vi "1.- FGV Serial.vi"(7 "VISA resource name":refnum<visa-resource-name>="COM3", 8 "error in (no error)":errorcluster, 10 "Command":string="H", 11 "Task":T1) -> (0 "error out":errorcluster, 2 "Receive buffer":string, 3 "return count":u32)   [LabVIEW 2014]
uses:
  control/FGV Serial Tasks.ctl
  <vilib>/Instr/_visa.llb/VISA Flush IO Buffer Mask.ctl
  <vilib>/Instr/_visa.llb/VISA Configure Serial Port (Instr).vi
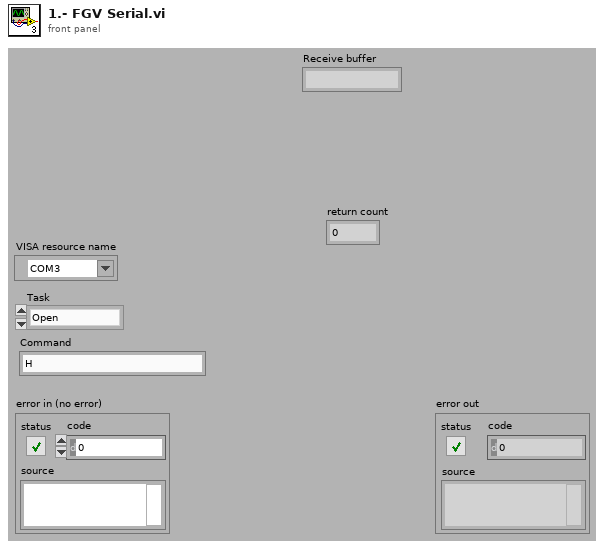
[diagram p1: front panel]
types:
  T1 = typedef "FGV Serial Tasks.ctl" = enum16{"Open", "Read", "Write", "Close", "Flush"}
  T2 = typedef "VISA Flush IO Buffer Mask.ctl" = u16
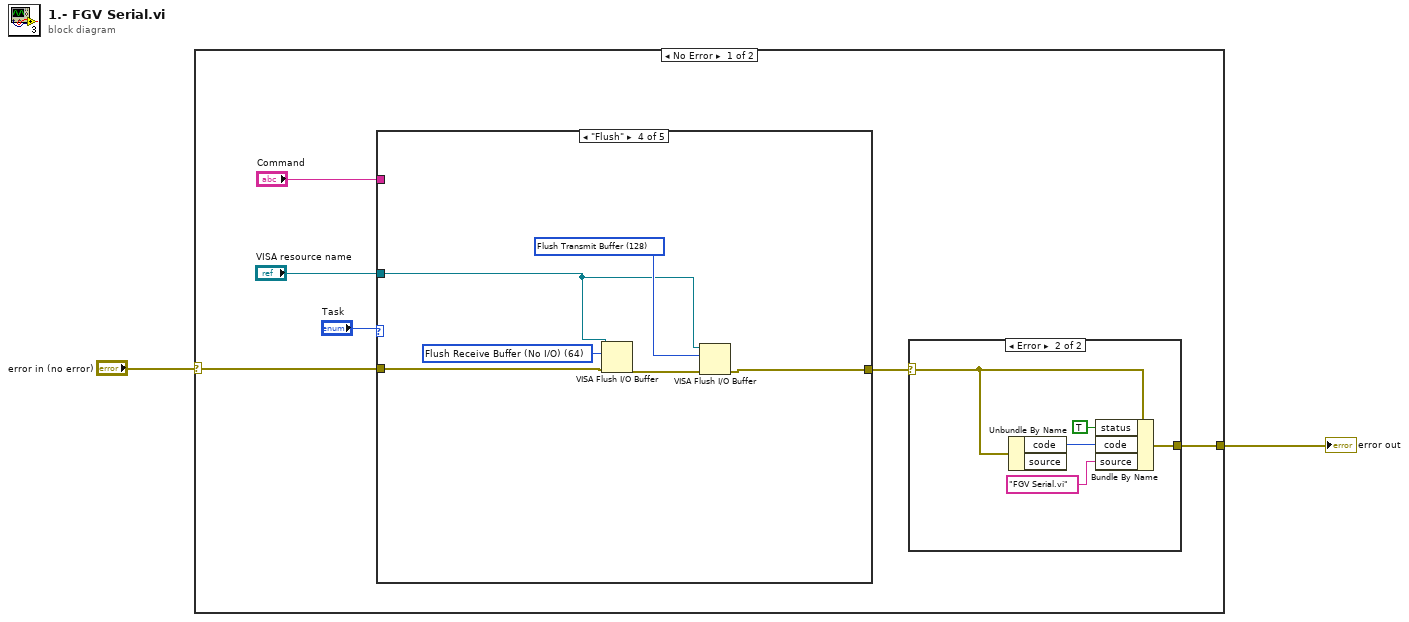
[diagram p0: block diagram]
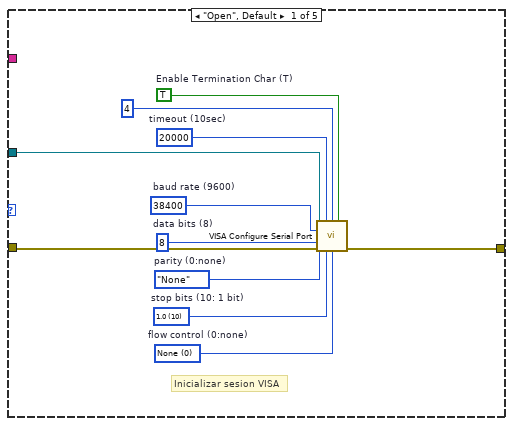
[diagram p3: hidden frame]
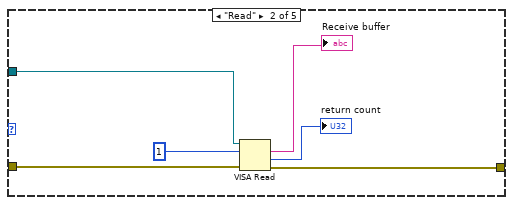
[diagram p4: hidden frame]
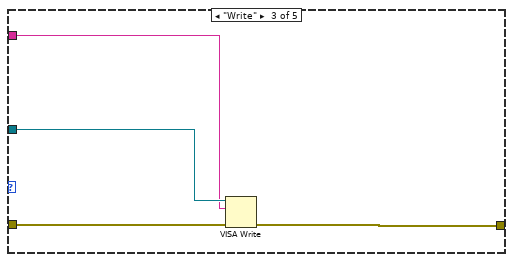
[diagram p5: hidden frame]
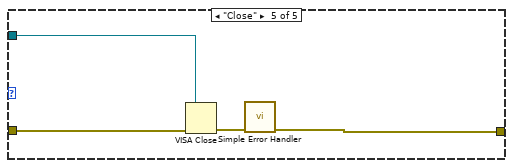
[diagram p6: hidden frame]
diagram:
  n1 = case shown="No Error" "error in (no error)" {
    selector: "error in (no error)" -> [w7 w46]
    tunnel: [w3 w46] -> w1
    frame No Error {
      n2 = case shown="\"Flush\"" "Task" {
        tunnel: "VISA resource name" -> [w18 w28 w33 w38 w42]
        tunnel: [w17 w31 w34 w36 w43] -> w4
        tunnel: w7 -> [w16 w27 w35 w41 w44]
        tunnel: "Command" -> [_ _ w32 _ _]
        frame "Open", Default {
          w23 = u16 0 items=["None", "XON/XOFF", "RTS/CTS", "XON/XOFF & RTS/CTS", "DTR/DSR", "XON/XOFF & DTR/DSR"]  # flow control (0:none)
          w22 = u16 10 items=["1.0"=10, "1.5"=15, "2.0"=20]  # stop bits (10: 1 bit)
          w21 = enum16{"None", "Odd", "Even", "Mark", "Space"}."None"  # parity (0:none)
          w20 = u16 8  # data bits (8)
          w19 = u32 38400  # baud rate (9600)
          w24 = u32 20000  # timeout (10sec)
          w25 = TRUE  # Enable Termination Char (T)
          # "Inicializar sesion VISA"
          n3 = call-poly "VISA Configure Serial Port"("VISA resource name"=w18, "timeout (10sec)"=w24, "termination char\n(0xA = '\\n' = LF)"=u8 4 ("termination char\n(0xA = '\\n' = LF)"), "Enable Termination\nChar (T)"=w25, "baud rate (9600)"=w19, "data bits (8)"=w20, "parity (0:none)"=w21, "error in (no error)"=w16, "stop bits (10: 1 bit)"=w22, "flow control (0:none)"=w23) -> ("error out"=w17:errorcluster)  [unwired: 4 in, 1 out]
        }
        frame "Read" {
          n4 = VISA Read(VISA resource name=w28, byte count=u32 1, error in (no error)=w27) -> (read buffer=→"Receive buffer":string, return count=→"return count":u32, error out=w31:errorcluster)  [unwired: 1 out]
        }
        frame "Write" {
          n5 = VISA Write(VISA resource name=w33, write buffer=w32, error in (no error)=w35) -> (error out=w34:errorcluster)  [unwired: 2 out]
        }
        frame "Flush" {
          w39 = T2 128 items=["Flush Receive Buffer"=16, "Write Transmit Buffer to Device"=32, "Flush Receive Buffer (No I/O)"=64, "Flush Transmit Buffer"=128] ("Mask")
          w40 = T2 64 items=["Flush Receive Buffer"=16, "Write Transmit Buffer to Device"=32, "Flush Receive Buffer (No I/O)"=64, "Flush Transmit Buffer"=128] ("Mask")
          n6 = VISA Flush I/O Buffer(VISA resource name=w38, mask (16)=w40, error in (no error)=w41) -> (error out=w37:errorcluster)  [unwired: 1 out]
          n7 = VISA Flush I/O Buffer(VISA resource name=w38, mask (16)=w39, error in (no error)=w37) -> (error out=w36:errorcluster)  [unwired: 1 out]
        }
        frame "Close" {
          n8 = VISA Close(VISA resource name=w42, error in (no error)=w44) -> (error out=w45:errorcluster)
          n9 = call <vilib>:"Simple Error Handler.vi"("error in (no error)"=w45) -> ("error out"=w43:errorcluster)  [unwired: 4 in, 4 out]
        }
      }
      n10 = case shown="Error" w4 {
        selector: w4 -> [w9 w13]
        tunnel: [w9 w12] -> w3
        frame No Error {
        }
        frame Error {
          n11 = Unbundle By Name(w13) -> ("code"=w14:i32)  [unwired: 1 out]
          n12 = Bundle By Name(cluster=w13, "status"=TRUE, "code"=w14, "source"="FGV Serial.vi") -> (w12:errorcluster)
        }
      }
    }
    frame Error {
    }
  }
  "error out" <- w1
